vi "Serial ESP8266 Tartget.vi"   [LabVIEW 2014]
doc: "The Serial - Monitoring GUI example shows best practices for a remote monitoring system with two VIs, one running on a host PC and the other running embedded in the Arduino compatible target. The example includes two-way serial communication between the host PC VI and the Arduino compatible target VI. This is the target VI taht generates a point by point sine wave that is charted by the host PC VI, writes the sine wave data points to the serial port and monitors the serial port for a potential pause/resume command to be sent by the host PC VI."
uses:
  <vilib>/Aledyne-TSXperts/Arduino Compatible Compiler for LabVIEW/Code Generator/Arduino APIs/Serial/Serial Settings.ctl
  <vilib>/Aledyne-TSXperts/Arduino Compatible Compiler for LabVIEW/Code Generator/Arduino APIs/Digital/PinDirection.ctl
  <vilib>/Aledyne-TSXperts/Arduino Compatible Compiler for LabVIEW/Arduino Compatible Compiler for LabVIEW.lvlib
types:
  T1 = typedef "Arduino Compatible Compiler for LabVIEW.lvlib/Serial Settings.ctl" = u16
  T2 = typedef "Arduino Compatible Compiler for LabVIEW.lvlib/PinDirection.ctl" = enum16{" INPUT", "OUTPUT", " INPUT_PULLUP"}
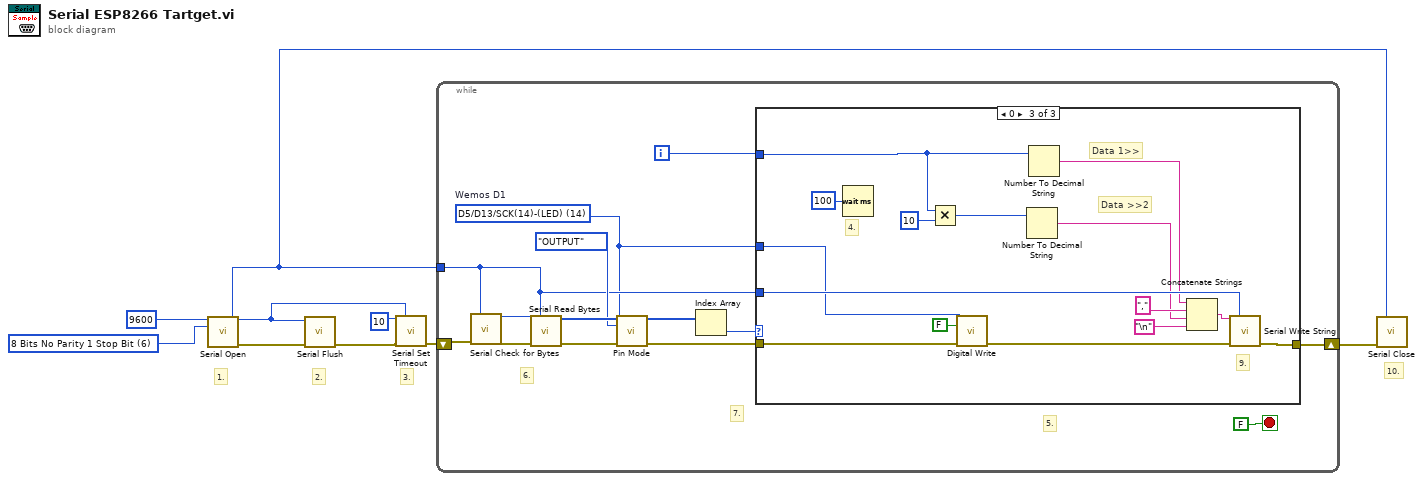
[diagram p0: block diagram]
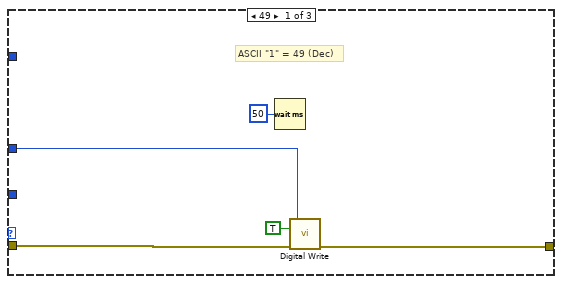
[diagram p2: hidden frame]
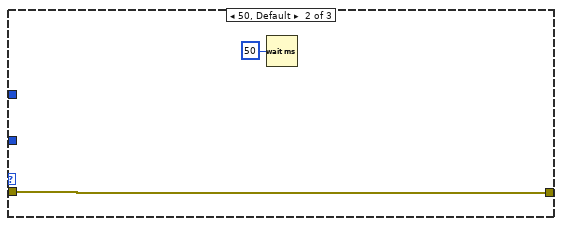
[diagram p3: hidden frame]
diagram:
  w6 = T1 6 items=["5 Bits No Parity 1 Stop Bit"=0, "6 Bits No Parity 1 Stop Bit"=2, "7 Bits No Parity 1 Stop Bit"=4, "8 Bits No Parity 1 Stop Bit"=6, "5 Bits No Parity 2 Stop Bits"=8, "6 Bits No Parity 2 Stop Bits"=10, "7 Bits No Parity 2 Stop Bits"=12, "8 Bits No Parity 2 Stop Bits"=14, "5 Bits Even Parity 1 Stop Bits"=32, "6 Bits Even Parity 1 Stop Bits"=34, "7 Bits Even Parity 1 Stop Bits"=36, "8 Bits Even Parity 1 Stop Bits"=38, "5 Bits Even Parity 2 Stop Bits"=40, "6 Bits Even Parity 2 Stop Bits"=42, "7 Bits Even Parity 2 Stop Bits"=44, "8 Bits Even Parity 2 Stop Bits"=46, "5 Bits Odd Parity 1 Stop Bits"=48, "6 Bits Odd Parity 1 Stop Bits"=50, "7 Bits Odd Parity 1 Stop Bits"=52, "8 Bits Odd Parity 1 Stop Bits"=54, "5 Bits Odd Parity 2 Stop Bits"=56, "6 Bits Odd Parity 2 Stop Bits"=58, "7 Bits Odd Parity 2 Stop Bits"=60, "8 Bits Odd Parity 2 Stop Bits"=62] ("Serial Settings")
  # "10."
  # "3."
  # "2."
  # "1."
  n1 = call <vilib>:"Serial Open.vi"("Speed"=u32 9600, "Serial Settings"=w6) -> ("Instance"=w3:u8, "error out"=w5:errorcluster)  [unwired: 12 in]
  n2 = call <vilib>:"Serial Flush.vi"("Instance"=w3, "error in (no error)"=w5) -> ("error out"=w4:errorcluster)  [unwired: 13 in]
  n3 = call <vilib>:"Serial Set Timeout.vi"("Timeout (ms)"=10, "Instance"=w3, "error in (no error)"=w4) -> ("error out"=w1:errorcluster)  [unwired: 12 in]
  n4 = while {
    tunnel: w3 -> [w10]
    shift-right: [w17] -> w7
    shift-left: w1 -> [w13]
    i -> [w18]
    stop <- FALSE stop-if-true
    w9 = u8 14 items=["D0-RX(3)"=3, "D1-TX(1)"=1, "D2(16)"=16, "D3/D15/SCL(5)"=5, "D4/D14/SDA(4)"=4, "D5/D13/SCK(14)-(LED)"=14, "D6/D12/MISO(12)"=12, "D7/D11/MOSI(13)"=13, "D8(0)"=0, "D9/TX1(2)"=2, "D10/SS (15)"=15, "ADC0,(17)"=17]  # Wemos D1
    # "7."
    # "6."
    # "5."
    n5 = call <vilib>:"Serial Check for Bytes.vi"("Instance"=w10, "error in (no error)"=w13) -> ("Bytes"=w11:i32, "error out"=w12:errorcluster)  [unwired: 12 in]
    n6 = call <vilib>:"Serial Read Bytes.vi"("Length"=w11, "Instance"=w10, "error in (no error)"=w12) -> ("Data"=w20:u8[], "error out"=w15:errorcluster)  [unwired: 10 in, 1 out]
    n7 = call <vilib>:"Pin Mode.vi"("pin"=w9, "direction"=PinDirection."OUTPUT", "error in (no error)"=w15) -> ("error out"=w14:errorcluster)  [unwired: 12 in]
    n8 = Index Array(array=w20) -> (element=w19:u8)  [unwired: 1 in]
    n9 = case shown="0" w19 {
      tunnel: [w24 w27 w43] -> w17
      tunnel: w14 -> [w25 w27 w32]
      tunnel: w10 -> [_ _ w42]
      tunnel: w18 -> [_ _ w36]
      tunnel: w9 -> [w23 _ w31]
      frame 49 {
        # "ASCII \"1\" = 49 (Dec)"
        n10 = Wait (ms)(milliseconds to wait=u32 50) -> ()  [unwired: 1 out]
        n11 = call <vilib>:"Digital Write.vi"("pin"=w23, "state"=TRUE, "error in (no error)"=w25) -> ("error out"=w24:errorcluster)  [unwired: 12 in]
      }
      frame 50, Default {
        n12 = Wait (ms)(milliseconds to wait=u32 50) -> ()  [unwired: 1 out]
      }
      frame 0 {
        # "Data >>2"
        # "Data 1>>"
        # "4."
        # "9."
        n13 = Wait (ms)(milliseconds to wait=u32 100) -> ()  [unwired: 1 out]
        n14 = Multiply(x=w36, y=10) -> (x*y=w30:i32)
        n15 = call <vilib>:"Digital Write.vi"("pin"=w31, "state"=FALSE, "error in (no error)"=w32) -> ("error out"=w34:errorcluster)  [unwired: 12 in]
        n16 = Number To Decimal String(number=w30) -> (decimal integer string=w29:string)  [unwired: 1 in]
        n17 = Number To Decimal String(number=w36) -> (decimal integer string=w37:string)  [unwired: 1 in]
        n18 = Concatenate Strings(w37, ",", w29, "\n" ("Line Feed Constant")) -> (w40:string)
        n19 = call <vilib>:"Serial Write String.vi"("String"=w40, "Instance"=w42, "error in (no error)"=w34) -> ("error out"=w43:errorcluster)  [unwired: 12 in]
      }
    }
  }
  n20 = call <vilib>:"Serial Close.vi"("Instance"=w3, "error in (no error)"=w7) -> ()  [unwired: 13 in, 1 out]
